vi "Check objects.vi"() -> ()   [LabVIEW 2021]
uses:
  HAL/Harware Abstraction/MultiIO/DMM.lvclass
  HAL/Concrete/Sim DMM/Sim DMM.lvclass
  C:/GitHub/OOP_OPC UA/Sequence/CodeModules/HAL/Harware Abstraction/MultiIO/DMM.lvclass
panel:
  out "Array 2":variant[](array[variant])
  out "Array":dbl[](array[numeric])
  in  "Setting":T1={"Resolution (Digits)"=5.5, "Current Source (Amps)"=0.001, "Range"=2.0, "Measurement Type"=enum."DC Volts"} {"Resolution (Digits)" items=["3 1/2"=3.5, "4 1/2"=4.5, "5 1/2"=5.5, "6 1/2"=6.5, "7 1/2"=7.5]; "Current Source (Amps)" items=["1uA"=1e-06, "10uA"=1e-05, "100uA"=0.0001, "1mA"=0.001]}
  out "Measurements":dbl
  in  "Instrument Ref":string="NI_DMM_4072"
  out "error out":errorcluster={"status"=TRUE, "code"=-1073807346, "source"="VISA Open in APS-7000 Series.lvlib:Initialize.vi->Concrete.lvlib:APS7050.lvclass:Initialise.vi->Check objects.vi"}
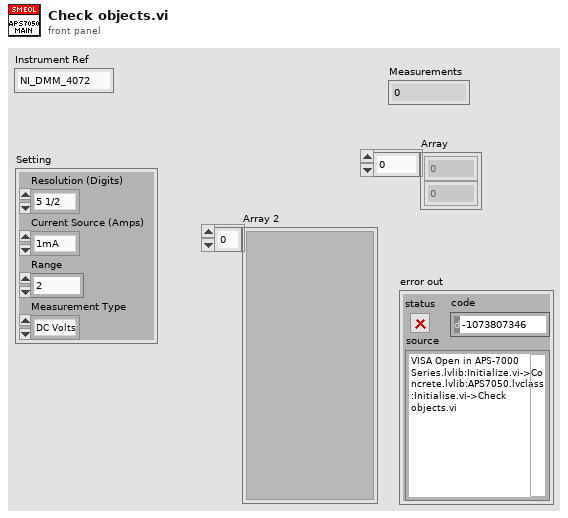
[diagram p1: front panel]
types:
  T1 = cluster{"Resolution (Digits)":dbl, "Current Source (Amps)":dbl, "Range":dbl, "Measurement Type":enum16{"DC Volts", "AC Volts", "DC Current", "AC Current", "2-wire Resistance", "4-wire Resistance", "Diode", "Frequency", "Period", "AC Volts DC Coupled", "Capacitance", "Inductance", "Temperature"}}
  T2 = typedef "MsgData.ctl" = cluster{"Message":string, "Data":variant}
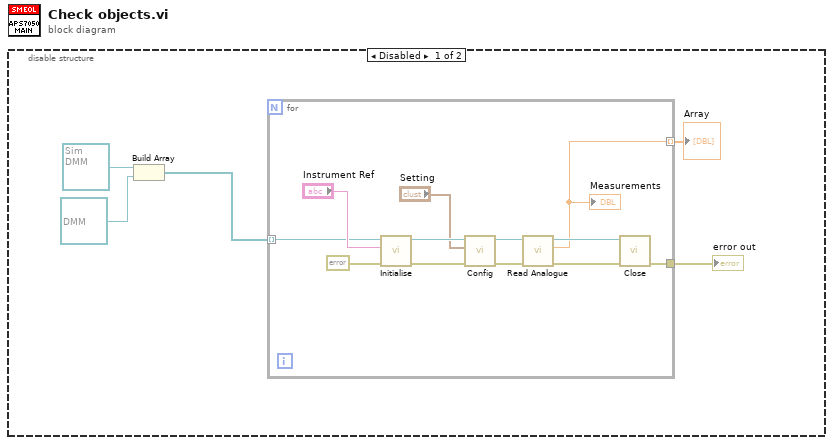
[diagram p0: block diagram]
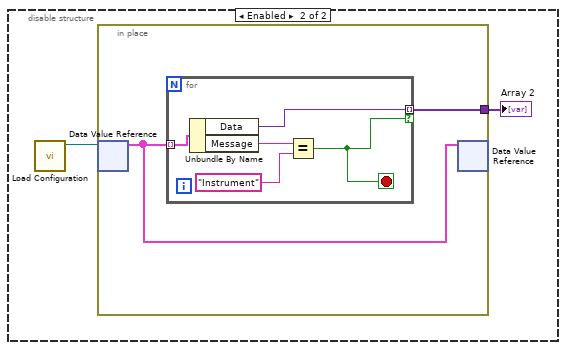
[diagram p2: hidden frame]
diagram:
  n1 = disable-structure shown="Disabled" {
    frame Disabled {
      n2 = Build Array(refnum<class "Sim DMM.lvclass"> refnum ("Concrete.lvlib:Sim DMM.lvclass"), refnum<class "DMM.lvclass"> refnum ("HAL.lvlib:DMM.lvclass")) -> (w2:refnum<class "DMM.lvclass">[])
      n3 = for {
        tunnel: [w17] -> w5
        tunnel: w2 -> [w7] mode=indexing
        tunnel: [w6] -> w1 mode=indexing
        n4 = call-dynamic "Initialise.vi"("error in (no error)"=errorcluster {"status"=FALSE, "code"=0, "source"=""}, "Instrument Ref"="Instrument Ref", "Instrument in"=w7) -> ("error out"=w11:errorcluster, "Instrument out"=w13:refnum<class "DMM.lvclass">)  [unwired: 7 in]
        n5 = call-dynamic "Config.vi"("error in (no error)"=w11, "Setting"="Setting", "DMM in"=w13) -> ("error out"=w10:errorcluster, "DMM out"=w12:refnum<class "DMM.lvclass">)  [unwired: 7 in]
        n6 = call-dynamic "Read Analogue.vi"("error in (no error)"=w10, "DMM in"=w12) -> ("error out"=w15:errorcluster, "Measurement"=w6:dbl, "DMM out"=w14:refnum<class "DMM.lvclass">)  [unwired: 7 in]
        "Measurements" <- w6
        n7 = call-dynamic "Close.vi"("error in (no error)"=w15, "Instrument in"=w14) -> ("error out"=w17:errorcluster)  [unwired: 8 in, 1 out]
      }
      "error out" <- w5
      "Array" <- w1
    }
    frame Enabled {
      n8 = call "Load Configuration.vi"() -> ("Config DVR"=w19:refnum<data-value>)  [unwired: 10 in, 1 out]
      n9 = in-place {
        in-place-border: [w21] -> w18
        n10 = in-place-dvr #1(w19) -> (w20:T2[])  [unwired: 1 out]
        n11 = for {
          tunnel: w20 -> [w26] mode=indexing
          tunnel: [w22] -> w21 mode=indexing if=w23
          stop <- w23 stop-if-true
          n12 = Unbundle By Name(w26) -> ("Data"=w22:variant, "Message"=w25:string)
          n13 = Equal?(x=w25, y="Instrument") -> (x = y?=w23:bool)
        }
        n14 = in-place-dvr #1(w20) -> ()  [unwired: 2 out]
      }
      "Array 2" <- w18
    }
  }
